vi "Create or Replace File.vi"(8 "error in":errorcluster, 10 "Log File Base Path":path) -> (0 "error out":errorcluster, 2 "File Path":path, 3 "Refnum out":refnum<k34>)   [LabVIEW 2026, in "Logger.lvlib"]
doc: "Create or replace the log file at the specified location.\n_____\nBased on DQMH Dev Tools: Project Template 7.1.2.1547."
uses:
  Logger.lvlib
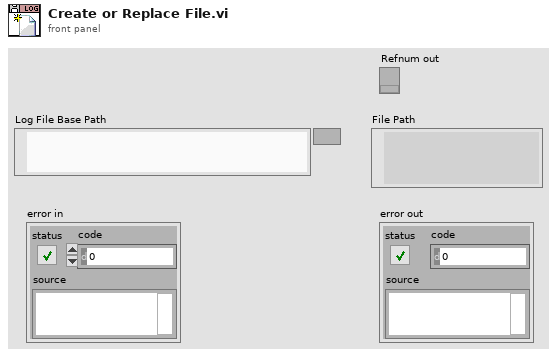
[diagram p1: front panel]
types:
  T1 = enum16{"open", "open or create", "create or replace", "create", "open (read-only)"}
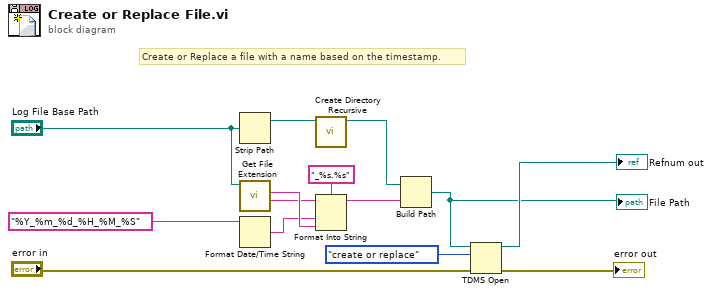
[diagram p0: block diagram]
diagram:
  # "Create or Replace a file with a name based on the timestamp."
  n1 = Strip Path(path="Log File Base Path") -> (stripped path=w2:path)  [unwired: 1 out]
  n2 = call <vilib>:"Get File Extension.vi"("file"="Log File Base Path") -> ("filename without extension"=w6:string, "lowercase file extension"=w9:string)  [unwired: 6 in, 3 out]
  n3 = Format Date/Time String(time format string (%c)="%Y_%m_%d_%H_%M_%S") -> (date/time string=w8:string)  [unwired: 2 in]
  n4 = call <vilib>:"Create Directory Recursive.vi"("directory"=w2) -> ("directory copy"=w1:path)  [unwired: 4 in, 2 out]
  n5 = Format Into String(format string="_%s.%s", initial string=w6, w8, w9) -> (resulting string=w10:string)  [unwired: 1 in, 1 out]
  n6 = Build Path(base path=w1, name or relative path=w10) -> (appended path=w3:path)
  "File Path" <- w3
  n7 = TDMS Open(8:"error in", 10:T1."create or replace" ("operation (0:open)"), 11:w3) -> (0:→"error out":errorcluster, 3:→"Refnum out":refnum<k34>)  [unwired: 4 in]
